vi "Status Get Temperature Units.vi"(5 "Retry Attempts (0)":i32 min=0, 7 "Unit Address (-1)":i32=-1, 8 "error in (no error)":errorcluster, 11 "VISA resource name (in)":refnum<visa-resource-name>) -> (0 "error out":errorcluster, 2 "Temperature Units":string, 3 "VISA resource name (out)":refnum<visa-resource-name>)   [LabVIEW 2020, in "Omega Platinum Series.lvlib"]
doc: "Retreives the current temperature units."
uses:
  <instrlib>/RxnRover/OmegaPlatinumSeriesDriver/Omega Platinum Series.lvlib
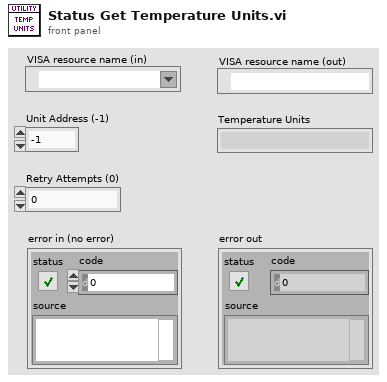
[diagram p1: front panel]
types:
  T1 = typedef "Omega Platinum Series.lvlib/Display Temperature Units.ctl" = enum16{"No units applied", "Celsius", "Fahrenheit"}
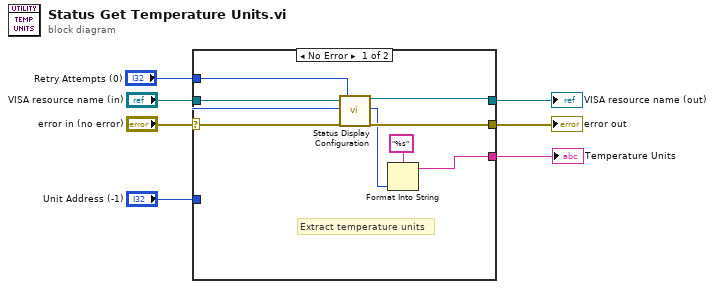
[diagram p0: block diagram]
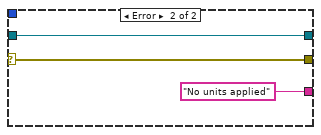
[diagram p2: hidden frame]
diagram:
  n1 = case shown="No Error" "error in (no error)" {
    selector: "error in (no error)" -> [w16 w19]
    tunnel: "Unit Address (-1)" -> [w10 _]
    tunnel: [w13 w19] -> w5
    tunnel: "VISA resource name (in)" -> [w12 w18]
    tunnel: [w11 w18] -> w3
    tunnel: [w14 "No units applied"] -> w2
    tunnel: "Retry Attempts (0)" -> [w8 _]
    frame No Error {
      # "Extract temperature units"
      n2 = call <instrlib>:"Status Display Configuration.vi"("VISA resource name (in)"=w12, "Unit Address (-1)"=w10, "error in (no error)"=w16, "Retry Attempts (0)"=w8) -> ("VISA resource name (out)"=w11:refnum<visa-resource-name>, "Temperature Units"=w9:T1, "error out"=w13:errorcluster)  [unwired: 10 in, 3 out]
      n3 = Format Into String(format string="%s", w9) -> (resulting string=w14:string)  [unwired: 2 in, 1 out]
    }
    frame Error {
    }
  }
  "error out" <- w5
  "VISA resource name (out)" <- w3
  "Temperature Units" <- w2
